vi "Convert String to Engine.vi"(6 "initialize (first call)":bool, 7 "transfer group id":i32, 8 "error in":errorcluster, 9 "string buffer":refnum<class "Buffer.lvclass">, 10 "engine buffer":refnum<class "Buffer.lvclass">, 11 "DSF buffer converter in":refnum<class "Default Buffer Converter.lvclass">) -> (0 "error out":errorcluster, 3 "DSF buffer converter out":refnum<class "Default Buffer Converter.lvclass">)   [LabVIEW 2019, in "DSF Core.lvlib" / "Default Buffer Converter.lvclass"]
uses:
  Default Buffer Converter.lvclass
  Classes/Buffer/Buffer.lvclass
  C:/Program Files (x86)/National Instruments/LabVIEW 2019/vi.lib/NI/Memory Manager/Classes/Pointer/Pointer.lvclass
  Default Buffer Converter.lvclass/Default Buffer Converter.ctl
  <vilib>/NI/Memory Manager/Classes/Pointer/Pointer.lvclass/Pointer.ctl
  <vilib>/NI/Memory Manager/Classes/Pointer/Write.vi
  <vilib>/NI/Memory Manager/Classes/Pointer/Write 1D U8.vi
  <vilib>/NI/Memory Manager/Classes/Pointer/Read.vi
  <vilib>/NI/Memory Manager/Classes/Pointer/Read 1D U8.vi
  Move String Block.vi
  <vilib>/NI/Memory Manager/Classes/Pointer/Write (No Check).vi
  <vilib>/NI/Memory Manager/Classes/Pointer/Write (No Check) 1D U8.vi
  <vilib>/NI/Memory Manager/Classes/Pointer/Check Move.vi
  <vilib>/NI/Memory Manager/Classes/Pointer/Read (No Check).vi
  <vilib>/NI/Memory Manager/Classes/Pointer/Read (No Check) 1D U8.vi
  VIs/Sizeof 1D.vi
  Classes/Buffer Converter/Convert String Data Type.vi
  <vilib>/NI/Memory Manager/Classes/Pointer/Get Address.vi
  <vilib>/NI/Memory Manager/Classes/Pointer/Check Null Pointer.vi
  <vilib>/NI/Memory Manager/Classes/Pointer/Check Count.vi
  <vilib>/NI/Memory Manager/Classes/Pointer/Check Bounds (Power of 2).vi
  VIs/Sizeof.vi
  <vilib>/NI/Memory Manager/Classes/Pointer/Errors.vi
  <vilib>/NI/Memory Manager/Classes/Pointer/Null Pointer.vi
  <vilib>/NI/Memory Manager/Classes/Pointer/Is Null.vi
  <vilib>/NI/Memory Manager/Classes/Pointer/Get Size.vi
  <vilib>/NI/Memory Manager/Classes/Pointer/Out of Bounds.vi
  <vilib>/NI/Memory Manager/Classes/Pointer/Check Bounds.vi
  <vilib>/NI/Memory Manager/Classes/Pointer/Create Error.vi
  <vilib>/NI/Memory Manager/VIs/Write String to Source.vi
  <vilib>/NI/Memory Manager/Classes/Pointer/Write Pointer Size to Error.vi
  <vilib>/NI/Memory Manager/VIs/Write Numeric to Source.vi
  <vilib>/NI/Memory Manager/VIs/Write Numeric Scalar to Source (Base10 U64).vi
  <vilib>/NI/Memory Manager/Classes/Pointer/Check Bounds (Pointer).vi
  <vilib>/NI/Memory Manager/Classes/Pointer/Check Bounds (Buffer).vi
  <vilib>/NI/Memory Manager/VIs/New Error Cluster.vi
  <vilib>/NI/Memory Manager/VIs/New Error Cluster (512B).vi
  <vilib>/NI/Memory Manager/VIs/Set Error Status.vi
  <vilib>/NI/Memory Manager/VIs/Set Error Code.vi
  <vilib>/NI/Memory Manager/VIs/Set Error Source.vi
  <vilib>/NI/Memory Manager/Constants/Constants.vi
  <vilib>/NI/Memory Manager/Constants/Library Name.vi
  <vilib>/NI/Memory Manager/Classes/Pointer/Pointer Error Info.vi
  <vilib>/NI/Memory Manager/Constants/Pointer Class Name.vi
  <vilib>/NI/Memory Manager/Classes/Pointer/Buffer Underflow.vi
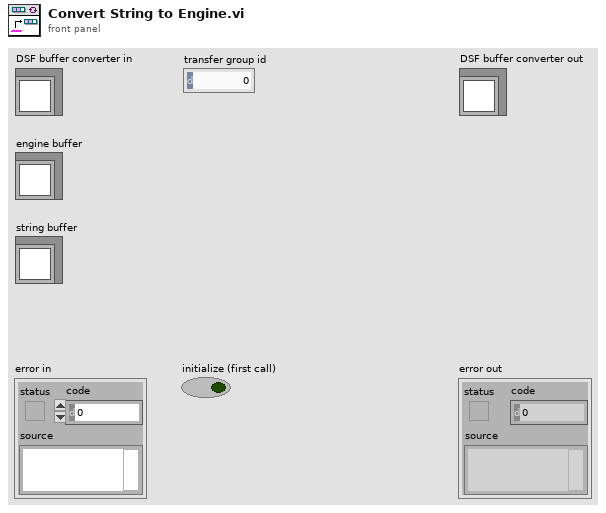
[diagram p1: front panel]
types:
  T1 = typedef "DSF Core.lvlib/Default Buffer Converter.lvclass/Conversion.ctl" = cluster{"conversion blocks":T2[]}
  T2 = typedef "DSF Core.lvlib/Default Buffer Converter.lvclass/Conversion Block.ctl" = cluster{"engine offset":u64, "engine data type":T3, "string offset":u64, "string data type":T3, "engine byte order":enum16{"big-endian, network order", "native, host order", "little-endian"}, "string byte order":enum16{"big-endian, network order", "native, host order", "little-endian"}, "count":u64}
  T3 = typedef "DSF Core.lvlib/DSF Data Type.ctl" = enum8{"Bool", "SGL", "DBL", "I8", "I16", "I32", "I64", "U8", "U16", "U32", "U64"}
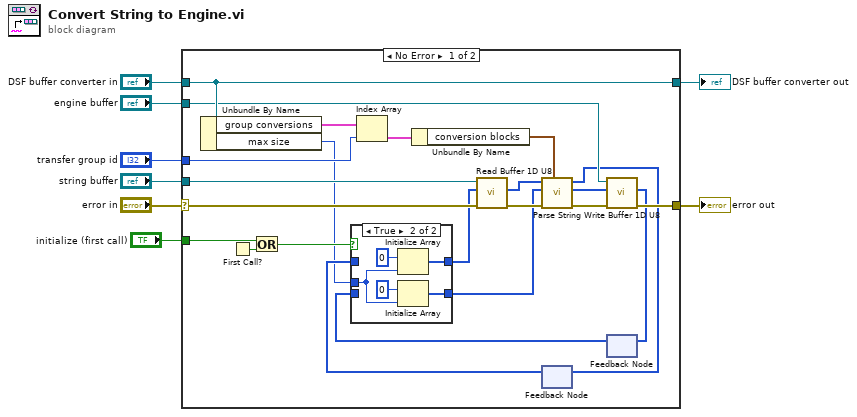
[diagram p0: block diagram]
diagram:
  n1 = case shown="No Error" "error in" {
    selector: "error in" -> [w18 w40]
    tunnel: [w17 w40] -> w7
    tunnel: [w29 w39] -> w5
    tunnel: "DSF buffer converter in" -> [w29 w39]
    tunnel: "transfer group id" -> [w28 _]
    tunnel: "string buffer" -> [w24 _]
    tunnel: "engine buffer" -> [w23 _]
    tunnel: "initialize (first call)" -> [w13 _]
    frame No Error {
      n2 = Unbundle By Name(w29) -> ("group conversions"=w31:T1[], "max size"=w9:u64)
      n3 = First Call?() -> (First Call?: T/F=w12:bool)
      n4 = Or(x=w13, y=w12) -> (x .or. y?=w11:bool)
      n5 = Index Array(array=w31, index=w28) -> (element=w30:T1)
      n6 = Unbundle By Name(w30) -> ("conversion blocks"=w14:T2[])
      n7 = feedback #1() -> (w20:u8[])  [unwired: 1 in]
      n8 = feedback #2() -> (w19:u8[])  [unwired: 1 in]
      n9 = case shown="True" w11 {
        tunnel: w9 -> [_ w34]
        tunnel: [w32 w37] -> w16
        tunnel: [w33 w35] -> w22
        tunnel: w19 -> [w33 _]
        tunnel: w20 -> [w32 _]
        frame False {
        }
        frame True {
          n10 = Initialize Array(u8 0 ("element"), w34) -> (w37:u8[])
          n11 = Initialize Array(u8 0 ("element"), w34) -> (w35:u8[])
        }
      }
      n12 = call "Read Buffer 1D U8.vi"("error in (no error)"=w18, "dst array in"=w16, "Buffer in"=w24) -> ("error out"=w27:errorcluster, "dst array out"=w25:u8[])  [unwired: 5 in, 2 out]
      n13 = call "Parse String.vi"("conversion blocks"=w14, "error in (no error)"=w27, "engine buffer in"=w22, "string buffer in"=w25) -> ("error out"=w26:errorcluster, "engine buffer out"=w21:u8[], "string buffer out"=w10:u8[])  [unwired: 5 in]
      n14 = feedback-in #1(w10) -> ()
      n15 = call "Write Buffer 1D U8.vi"("error in (no error)"=w26, "src array in"=w21, "Buffer in"=w23) -> ("error out"=w17:errorcluster, "src array out"=w15:u8[])  [unwired: 5 in, 2 out]
      n16 = feedback-in #2(w15) -> ()
    }
    frame Error {
    }
  }
  "error out" <- w7
  "DSF buffer converter out" <- w5
